vi "XY Go.vi"(4 "Increment?":bool, 6 "return immediately":bool, 8 "error in (no error)":errorcluster, 9 "Speed":dbl, 10 "XY In":dbl[](array[numeric]), 11 "Gantry In":refnum<k24>) -> (0 "error out":errorcluster, 2 "XY Out":dbl[](array[numeric]), 3 "Gantry Out":refnum<k24>)   [LabVIEW 2021, in "A3200.lvclass"]
uses:
  A3200.lvclass
  C:/Program Files (x86)/Aerotech/A3200/LabVIEW/2010/Bin/Aerotech.A3200.dll
  Program Files (x86)/Aerotech/A3200/LabVIEW/2010/Bin/Aerotech.A3200.dll
  Drivers/Aerotech A3200/Aerotech.lvlib
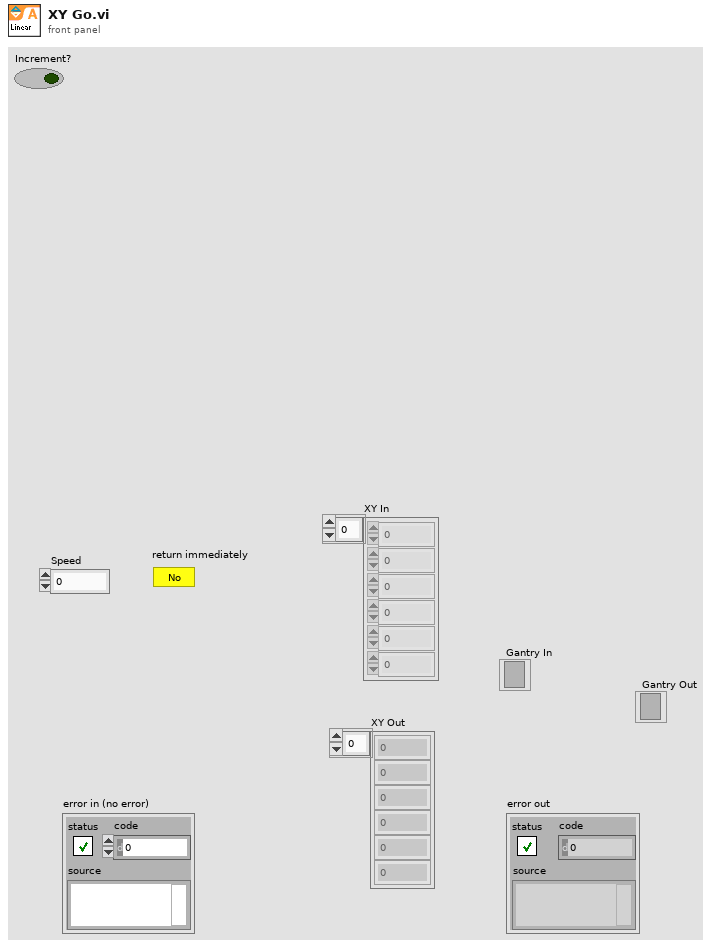
[diagram p1: front panel]
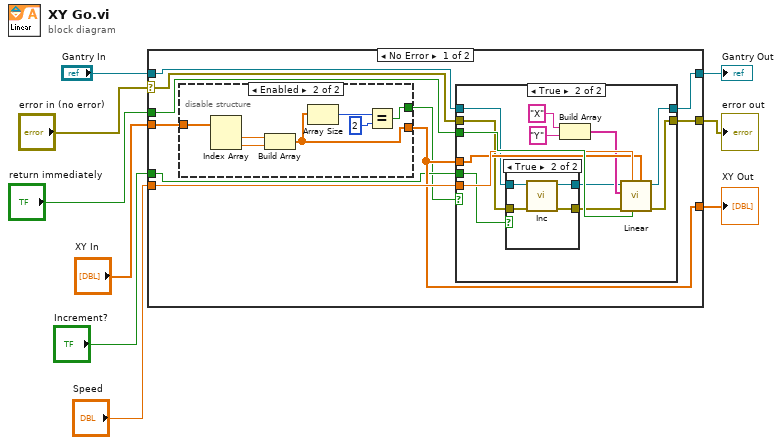
[diagram p0: block diagram]
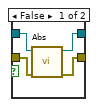
[diagram p3: hidden frame]
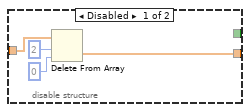
[diagram p4: hidden frame]
diagram:
  n1 = case shown="No Error" "error in (no error)" {
    selector: "error in (no error)" -> [w12 w56]
    tunnel: [w18 w56] -> w8
    tunnel: [w19 w55] -> w6
    tunnel: "Gantry In" -> [w11 w55]
    tunnel: "return immediately" -> [w17 _]
    tunnel: [w14 w54] -> w4
    tunnel: "XY In" -> [w15 w54]
    tunnel: "Speed" -> [w16 _]
    tunnel: "Increment?" -> [w13 _]
    frame No Error {
      n2 = disable-structure shown="Enabled" {
        disable-tunnel: w15 -> [w46 w53]
        disable-tunnel: [w43 w50] -> w14
        disable-tunnel: [_ w47] -> w10
        frame Disabled {
          n3 = Delete From Array(array=w46, length=2, index=0) -> (deleted portion=w43:dbl[])  [unwired: 1 out]
        }
        frame Enabled {
          n4 = Index Array(array=w53) -> (element #1=w52:dbl, element #2=w51:dbl)  [unwired: 2 in]
          n5 = Build Array(w52, w51) -> (w50:dbl[])
          n6 = Array Size(array=w50) -> (size(s)=w49:i32)
          n7 = Equal?(x=w49, y=2) -> (x = y?=w47:bool)
        }
      }
      n8 = case shown="True" w10 {
        tunnel: [w21 w34] -> w19
        tunnel: [w20 w22] -> w18
        tunnel: w17 -> [_ w33]
        tunnel: w16 -> [_ w32]
        tunnel: w14 -> [_ w31]
        tunnel: w13 -> [_ w30]
        tunnel: w12 -> [w20 w29]
        tunnel: w11 -> [w21 w28]
        frame False {
        }
        frame True {
          n9 = case shown="True" w30 {
            tunnel: w29 -> [w38 w40]
            tunnel: w28 -> [w37 w42]
            tunnel: [w36 w39] -> w24
            tunnel: [w35 w41] -> w23
            frame False {
              n10 = call "Abs.vi"("error in (no error)"=w38, "controller in"=w37) -> ("error out"=w36:errorcluster, "controller out"=w35:refnum<k24>)  [unwired: 8 in]
            }
            frame True {
              n11 = call "Inc.vi"("error in (no error)"=w40, "controller in"=w42) -> ("error out"=w39:errorcluster, "controller out"=w41:refnum<k24>)  [unwired: 8 in]
            }
          }
          n12 = Build Array("X" ("format string"), "Y" ("format string")) -> (w25:string[])
          n13 = call "Linear.vi"("distances"=w31, "return immediately"=w33, "speed"=w32, "error in (no error)"=w24, "axis names"=w25, "controller in"=w23) -> ("error out"=w22:errorcluster, "controller out"=w34:refnum<k24>)  [unwired: 4 in]
        }
      }
    }
    frame Error {
    }
  }
  "error out" <- w8
  "Gantry Out" <- w6
  "XY Out" <- w4
